vi "interface.vi"() -> ()   [LabVIEW 2010]
uses:
  Global 1.vi
  <vilib>/Instr/_visa.llb/VISA Configure Serial Port (Instr).vi
  <vilib>/Utility/file.llb/Write To Spreadsheet File (I64).vi
panel:
  in  "lecture":string
  in  "send_speed":bool
  in  "Speed":u32=1 min=1 max=200 step=10
  out "connected-led":bool
  in  "disconnect/connect":bool
  out "Waveform Graph":i32[](graph)
  in  "Path:":path
  in  "Save":bool
  in  "invert":bool
  in  "reset":bool
  in  "Run":bool
  out "?":errorcluster
  in  "PORT:":refnum<visa-resource-name>
  # "Horno-CS  control system"
  # "GICM"
  # "daniel.estrada1@udea.edu.co"
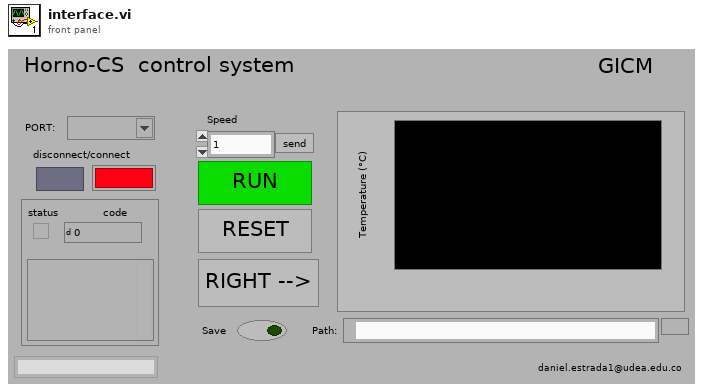
[diagram p1: front panel]
types:
  T1 = enum8{"Enabled", "Disabled", "Disabled and Grayed Out"}
  T2 = enum16{"open", "replace", "create", "open or create", "replace or create", "replace or create with confirmation"}
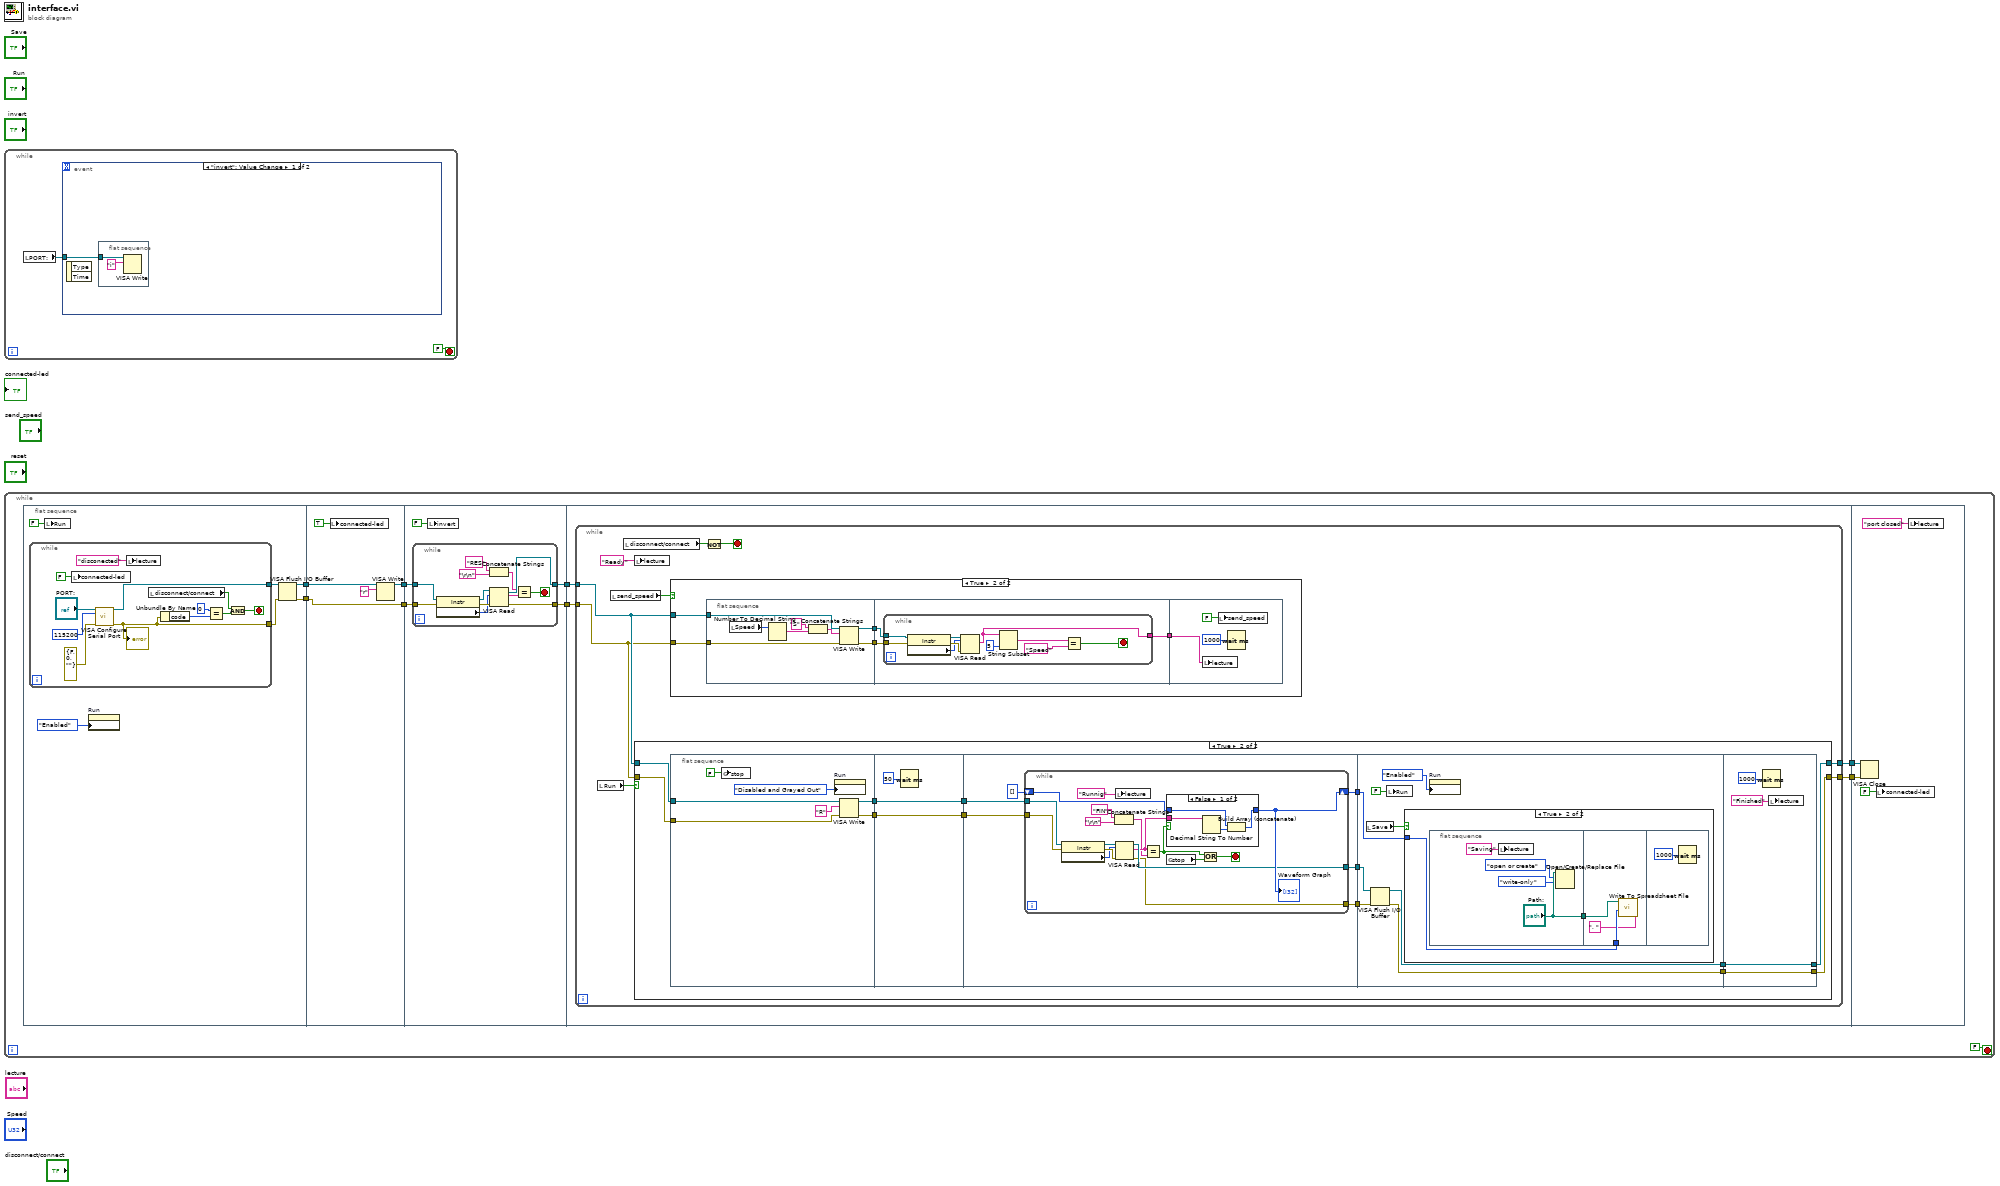
[diagram p0: block diagram]
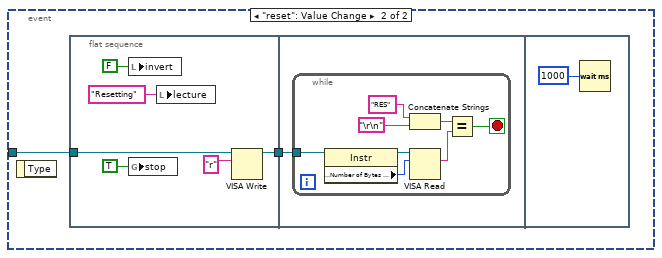
[diagram p2: hidden frame]
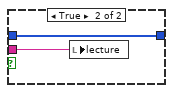
[diagram p5: hidden frame]
diagram:
  n1 = while {
    stop <- FALSE stop-if-true
    n2 = local read "PORT:"() -> (w1:refnum<visa-resource-name>)
    n3 = event shown="[0] \"invert\": Value Change" {
      selector: _ -> [_ _]
      dyn-events: _ -> [_ _]
      timeout: _ -> [_ _]
      tunnel: w1 -> [w3 w6]
      event "invert": Value Change {
        n4 = event-data() -> ()  [unwired: 1 in, 2 out]
        n5 = flat-sequence {
          tunnel: w3 -> [w5]
          frame #0 {
            n6 = VISA Write(VISA resource name=w5, write buffer="i") -> ()  [unwired: 1 in, 3 out]
          }
        }
      }
      event "reset": Value Change {
        n7 = event-data() -> ()  [unwired: 1 in, 1 out]
        n8 = flat-sequence {
          tunnel: [w13] -> w7
          tunnel: w6 -> [w9]
          tunnel: w7 -> [w14]
          frame #0 {
            n9 = local write "invert"(FALSE ("invert")) -> ()
            n10 = global write "Global 1.vi" "stop"(TRUE ("stop")) -> ()
            n11 = local write "lecture"("Resetting" ("lecture")) -> ()
            n12 = VISA Write(VISA resource name=w9, write buffer="r") -> (VISA resource name out=w13:refnum<visa-resource-name>)  [unwired: 1 in, 2 out]
          }
          frame #1 {
            n13 = while {
              tunnel: w14 -> [w21]
              stop <- w15 stop-if-true
              n14 = property class="Instr"(reference=w21) -> (reference out=w22:refnum<visa-resource-name>, "Serial Settings:Number of Bytes at Serial Port"=w20:u32)  [unwired: 1 in, 1 out]
              n15 = Concatenate Strings("RES" ("string"), "\r\n") -> (w19:string)
              n16 = VISA Read(VISA resource name=w22, byte count=w20) -> (read buffer=w16:string)  [unwired: 1 in, 3 out]
              n17 = Equal?(x=w19, y=w16) -> (x = y?=w15:bool)
            }
          }
          frame #2 {
            n18 = Wait (ms)(milliseconds to wait=u32 1000) -> ()  [unwired: 1 out]
          }
        }
      }
    }
  }
  n19 = while {
    stop <- FALSE stop-if-true
    n20 = flat-sequence {
      tunnel: [w38] -> w27
      tunnel: [w37] -> w24
      tunnel: [w55] -> w26
      tunnel: [w54] -> w25
      tunnel: w24 -> [w54]
      tunnel: w27 -> [w51]
      tunnel: [w59] -> w29
      tunnel: [w58] -> w28
      tunnel: w26 -> [w60]
      tunnel: w25 -> [w57]
      tunnel: [w74] -> w32
      tunnel: [w73] -> w31
      tunnel: w29 -> [w76]
      tunnel: w28 -> [w75]
      tunnel: w32 -> [w192]
      tunnel: w31 -> [w191]
      frame #0 {
        n21 = while {
          tunnel: [w46] -> w36
          tunnel: [w44] -> w35
          stop <- w41 stop-if-true
          n22 = local write "connected-led"(FALSE ("connected-led")) -> ()
          n23 = call-poly "VISA Configure Serial Port"("VISA resource name"="PORT:", "baud rate (9600)"=u32 115200, "error in (no error)"=errorcluster {"status"=FALSE, "code"=0, "source"=""}) -> ("VISA resource name out"=w46:refnum<visa-resource-name>, "error out"=w44:errorcluster)  [unwired: 11 in]
          "?" <- w44
          n24 = local write "lecture"("disconected" ("lecture")) -> ()
          n25 = local read "disconnect/connect"() -> (w47:bool)
          n26 = Unbundle By Name(w44) -> ("code"=w43:i32)
          n27 = Equal?(x=0, y=w43) -> (x = y?=w40:bool)
          n28 = And(x=w47, y=w40) -> (x .and. y?=w41:bool)
        }
        n29 = local write "Run"(FALSE ("Run")) -> ()
        n30 = property on="Run" class="Bool (strict)"("DisabledEnum"=T1."Enabled" ("Disabled")) -> ()  [unwired: 2 in, 2 out]
        n31 = VISA Flush I/O Buffer(VISA resource name=w36, error in (no error)=w35) -> (VISA resource name out=w38:refnum<visa-resource-name>, error out=w37:errorcluster)  [unwired: 1 in]
      }
      frame #1 {
        n32 = local write "connected-led"(TRUE ("connected-led")) -> ()
        n33 = VISA Write(VISA resource name=w51, write buffer="r") -> (VISA resource name out=w55:refnum<visa-resource-name>)  [unwired: 1 in, 2 out]
      }
      frame #2 {
        n34 = while {
          tunnel: w60 -> [w71]
          tunnel: [w69] -> w59
          tunnel: [w68] -> w58
          tunnel: w57 -> [w67]
          stop <- w61 stop-if-true
          n35 = property class="Instr"(reference=w71, error in=w67) -> (reference out=w70:refnum<visa-resource-name>, error out=w72:errorcluster, "Serial Settings:Number of Bytes at Serial Port"=w66:u32)
          n36 = Concatenate Strings("RES" ("string"), "\r\n") -> (w65:string)
          n37 = VISA Read(VISA resource name=w70, byte count=w66, error in (no error)=w72) -> (VISA resource name out=w69:refnum<visa-resource-name>, read buffer=w64:string, error out=w68:errorcluster)  [unwired: 1 out]
          n38 = Equal?(x=w65, y=w64) -> (x = y?=w61:bool)
        }
        n39 = local write "invert"(FALSE ("invert")) -> ()
      }
      frame #3 {
        n40 = while {
          tunnel: w76 -> [w83]
          tunnel: w75 -> [w82]
          tunnel: [w79] -> w74
          tunnel: [w78] -> w73
          stop <- w81 stop-if-true
          n41 = local read "Run"() -> (w85:bool)
          n42 = local read "send_speed"() -> (w84:bool)
          n43 = local read "disconnect/connect"() -> (w80:bool)
          n44 = local write "lecture"("Ready" ("lecture")) -> ()
          n45 = case shown="True" w85 {
            tunnel: w83 -> [w116 w129]
            tunnel: w82 -> [w115 w128]
            tunnel: [w116 w127] -> w79
            tunnel: [w115 w125] -> w78
            frame False {
            }
            frame True {
              n46 = flat-sequence {
                tunnel: w128 -> [w133]
                tunnel: w129 -> [w134]
                tunnel: [w131] -> w122
                tunnel: [w130] -> w120
                tunnel: w122 -> [w139]
                tunnel: [w139] -> w121
                tunnel: w120 -> [w138]
                tunnel: [w138] -> w119
                tunnel: [w142] -> w126
                tunnel: [w141] -> w124
                tunnel: [w140] -> w123
                tunnel: w121 -> [w145]
                tunnel: w119 -> [w144]
                tunnel: w126 -> [w173]
                tunnel: w124 -> [w172]
                tunnel: w123 -> [w175]
                tunnel: [w170] -> w118
                tunnel: [w171] -> w117
                tunnel: [w189] -> w125
                tunnel: [w190] -> w127
                tunnel: w118 -> [w190]
                tunnel: w117 -> [w189]
                frame #0 {
                  n47 = global write "Global 1.vi" "stop"(FALSE ("stop")) -> ()
                  n48 = property on="Run" class="Bool (strict)"("DisabledEnum"=T1."Disabled and Grayed Out" ("Disabled")) -> ()  [unwired: 2 in, 2 out]
                  n49 = VISA Write(VISA resource name=w134, write buffer="R", error in (no error)=w133) -> (VISA resource name out=w131:refnum<visa-resource-name>, error out=w130:errorcluster)  [unwired: 1 out]
                }
                frame #1 {
                  n50 = Wait (ms)(milliseconds to wait=u32 50) -> ()  [unwired: 1 out]
                }
                frame #2 {
                  n51 = while {
                    tunnel: w145 -> [w162]
                    tunnel: w144 -> [w161]
                    shift-right: [w157] -> w140
                    shift-left: i32[] [] -> [w158]
                    tunnel: [w156] -> w142
                    tunnel: [w155] -> w141
                    stop <- w153 stop-if-true
                    n52 = property class="Instr"(reference=w162, error in=w161) -> (reference out=w160:refnum<visa-resource-name>, error out=w159:errorcluster, "Serial Settings:Number of Bytes at Serial Port"=w147:u32)
                    n53 = Concatenate Strings("FIN" ("y"), "\r\n") -> (w150:string)
                    n54 = local write "lecture"("Runnig" ("lecture")) -> ()
                    n55 = VISA Read(VISA resource name=w160, byte count=w147, error in (no error)=w159) -> (VISA resource name out=w156:refnum<visa-resource-name>, read buffer=w151:string, error out=w155:errorcluster)  [unwired: 1 out]
                    n56 = Equal?(x=w151, y=w150) -> (x = y?=w152:bool)
                    n57 = case shown="False" w152 {
                      tunnel: w151 -> [w166 w167]
                      tunnel: w158 -> [w163 w168]
                      tunnel: [w164 w168] -> w157
                      frame False {
                        n58 = Decimal String To Number(string=w166) -> (number=w165:i32)  [unwired: 2 in, 1 out]
                        n59 = Build Array (concatenate)(w163, w165) -> (w164:i32[])
                      }
                      frame True {
                        n60 = local write "lecture"(w167) -> ()
                      }
                    }
                    "Waveform Graph" <- w157
                    n61 = global read "Global 1.vi" "stop"() -> (w154:bool)
                    n62 = Or(x=w152, y=w154) -> (x .or. y?=w153:bool)
                  }
                }
                frame #3 {
                  n63 = local read "Save"() -> (w176:bool)
                  n64 = VISA Flush I/O Buffer(VISA resource name=w173, error in (no error)=w172) -> (VISA resource name out=w170:refnum<visa-resource-name>, error out=w171:errorcluster)  [unwired: 1 in]
                  n65 = local write "Run"(FALSE ("Run")) -> ()
                  n66 = case shown="True" w176 {
                    tunnel: w175 -> [_ w177]
                    frame False {
                    }
                    frame True {
                      n67 = flat-sequence {
                        tunnel: ["Path:"] -> w178
                        tunnel: w178 -> [w185]
                        tunnel: w177 -> [w184]
                        frame #0 {
                          n68 = local write "lecture"("Saving" ("lecture")) -> ()
                          n69 = Open/Create/Replace File(file path (use dialog)="Path:", operation (0:open)=T2."open or create", access (0:read/write)=enum16{"read/write", "read-only", "write-only"}."write-only") -> ()  [unwired: 3 in, 3 out]
                        }
                        frame #1 {
                          n70 = call-poly <vilib>:"Write To Spreadsheet File.vi"("delimiter (\\t)"=", " ("delimiter (\\t)"), "1D data"=w184, "file path (dialog if empty)"=w185) -> ()  [unwired: 5 in, 1 out]
                        }
                        frame #2 {
                          n71 = Wait (ms)(milliseconds to wait=u32 1000) -> ()  [unwired: 1 out]
                        }
                      }
                    }
                  }
                  n72 = property on="Run" class="Bool (strict)"("DisabledEnum"=T1."Enabled" ("Disabled")) -> ()  [unwired: 2 in, 2 out]
                }
                frame #4 {
                  n73 = Wait (ms)(milliseconds to wait=u32 1000) -> ()  [unwired: 1 out]
                  n74 = local write "lecture"("Finished" ("lecture")) -> ()
                }
              }
            }
          }
          n75 = case shown="True" w84 {
            tunnel: w82 -> [_ w90]
            tunnel: w83 -> [_ w89]
            frame False {
            }
            frame True {
              n76 = flat-sequence {
                tunnel: [w98] -> w88
                tunnel: [w97] -> w87
                tunnel: w90 -> [w91]
                tunnel: w89 -> [w92]
                tunnel: w88 -> [w101]
                tunnel: w87 -> [w100]
                tunnel: [w99] -> w86
                tunnel: w86 -> [w113]
                frame #0 {
                  n77 = local read "Speed"() -> (w96:u32)
                  n78 = Number To Decimal String(number=w96) -> (decimal integer string=w95:string)  [unwired: 1 in]
                  n79 = Concatenate Strings("S" ("string"), w95) -> (w94:string)
                  n80 = VISA Write(VISA resource name=w92, write buffer=w94, error in (no error)=w91) -> (VISA resource name out=w98:refnum<visa-resource-name>, error out=w97:errorcluster)  [unwired: 1 out]
                }
                frame #1 {
                  n81 = while {
                    tunnel: w101 -> [w109]
                    tunnel: w100 -> [w108]
                    tunnel: [w102] -> w99
                    stop <- w106 stop-if-true
                    n82 = property class="Instr"(reference=w109, error in=w108) -> (reference out=w111:refnum<visa-resource-name>, error out=w110:errorcluster, "Serial Settings:Number of Bytes at Serial Port"=w107:u32)
                    n83 = VISA Read(VISA resource name=w111, byte count=w107, error in (no error)=w110) -> (read buffer=w102:string)  [unwired: 3 out]
                    n84 = String Subset(string=w102, length (rest)=5 ("length (rest)")) -> (substring=w104:string)  [unwired: 1 in]
                    n85 = Equal?(x=w104, y="Speed" ("string")) -> (x = y?=w106:bool)
                  }
                }
                frame #2 {
                  n86 = local write "lecture"(w113) -> ()
                  n87 = local write "send_speed"(FALSE ("send_speed")) -> ()
                  n88 = Wait (ms)(milliseconds to wait=u32 1000) -> ()  [unwired: 1 out]
                }
              }
            }
          }
          n89 = Not(x=w80) -> (.not. x?=w81:bool)
        }
      }
      frame #4 {
        n90 = VISA Close(VISA resource name=w192, error in (no error)=w191) -> ()  [unwired: 1 out]
        n91 = local write "connected-led"(FALSE ("connected-led")) -> ()
        n92 = local write "lecture"("port closed" ("lecture")) -> ()
      }
    }
  }
